vi "Puff_Dose.vi"() -> (5 "Plug in titles":string[](array[string]), 7 "Plug in values":string[](array[string]))   [LabVIEW 2015]
uses:
  Controls/Post_Process.ctl
  <vilib>/Analysis/baseanly.llb/Mean (DBL).vi
  Globals/Meas_global.vi
  Globals/Plug_in_data_global.vi
  <vilib>/Analysis/NI_AALBase.lvlib
panel:
  out "Active Trace length":i32
  out "Background time used (s)":dbl
  out "Delta T":dbl
  out "Min Dose":dbl
  out "Stats Names":string[](array[string])
  out "Stats values":string[](array[string])
  in  "File Extension":string=".xls"
  in  "Save Puff file":bool
  out "Bkgnd value (ppm)":dbl format="%0.2f"
  out "Array":dbl[][](array[numeric])
  out "Puff Number":i32=51
  out "XY Graph":cluster{"Time (s)":dbl[], "Eng Values":dbl[]}[](graph)
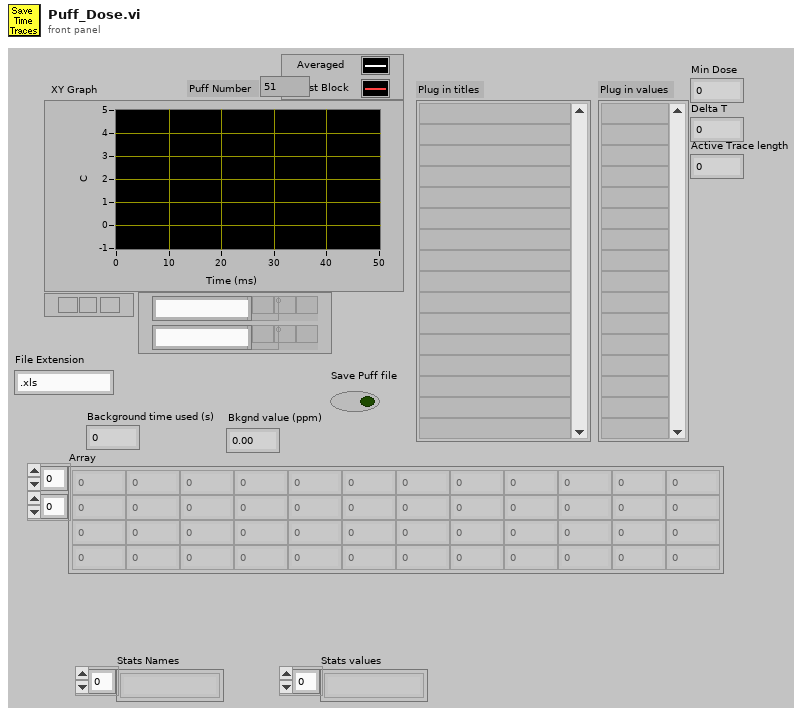
[diagram p1: front panel]
types:
  T1 = typedef "Analysis_info_cluster.ctl" = cluster{"Colour":u32, "Inst type":T2, "Inst name":string, "Symbol":string, "Code name":string, "Extra Info":string, "Inst Array":T3, "Extra Titles":string[], "Extra Values":string[], "U":dbl, "u^2":dbl, "u^3":dbl, "u^4":dbl, "Skew_u":dbl, "Kurt_u":dbl, "Sd Error in Mean":dbl, "% u'/U":dbl, "X":dbl, "Y":dbl, "Z":dbl, "Timescale integral to 25%":dbl, "Sd Error in Variance":dbl, "Calib File":path, "Calib Constants":dbl[], "Output Position":bool, "Full Stats":bool, "Av Sampling Rate":dbl, "Av No of Samples":dbl, "Total Meas Time (s)":dbl, "ADAM Ch Name":string}
  T2 = typedef "Inst_type.ctl" = enum16{"Propeller anemometer", "Raw voltage", "Pressure Transducer", "Pitot-static tube", "Preston tube", "Hot wire", "Cross wire 1", "Cross wire 2", "Generic Linear", "Generic Polynomial", "Generic BackPoly", "Fast FID", "Thermocouple", "Cold wire", "Pulsed Wire", "LDA Vel", "LDA Tran time", "LDA Arr time", "Microphone"}
  T3 = typedef "Instrument_Array.ctl" = enum16{"PWA", "LDA", "Analogue"}
  T4 = typedef "Post_Process.ctl" = enum16{"Take New Data", "Post Process Raw Data File"}
  T5 = enum16{"Save no data", "Save data in new files", "Save data in existing files"}
  T6 = typedef "Time_Trace_Cluster.ctl" = cluster{"Weighting":dbl[], "Time (s)":dbl[], "Voltage":dbl[], "Eng Values":dbl[]}
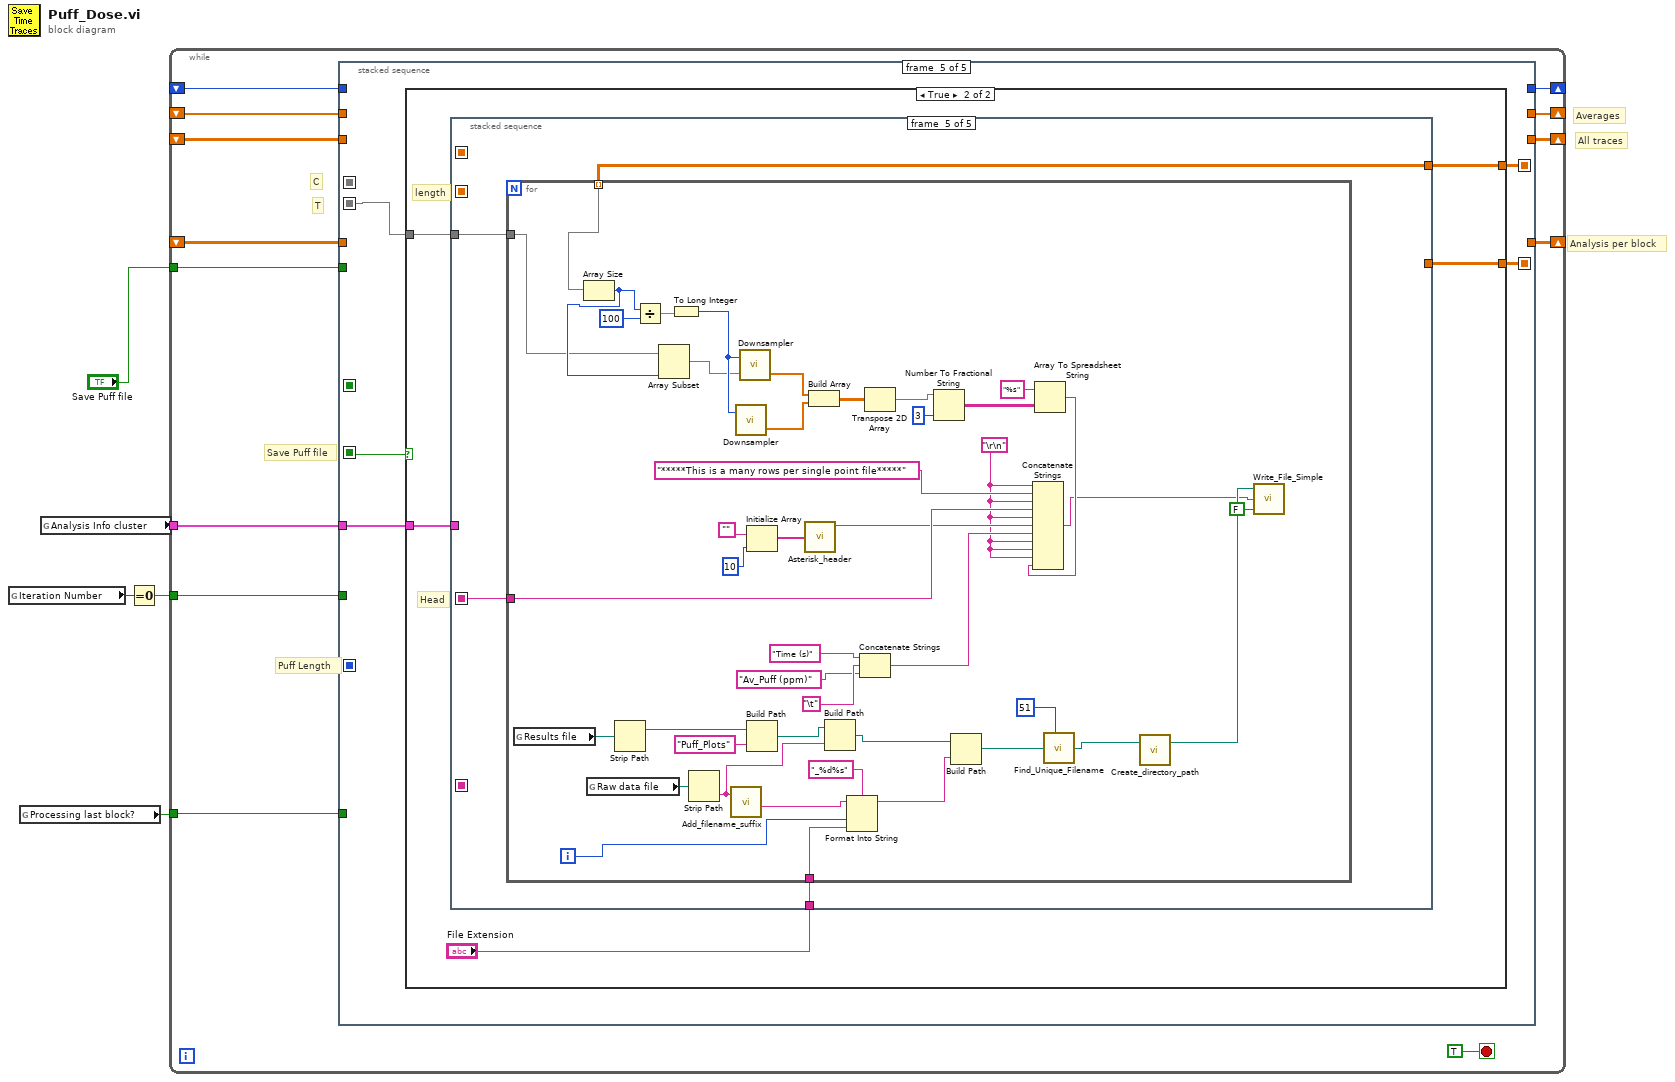
[diagram p0: block diagram]
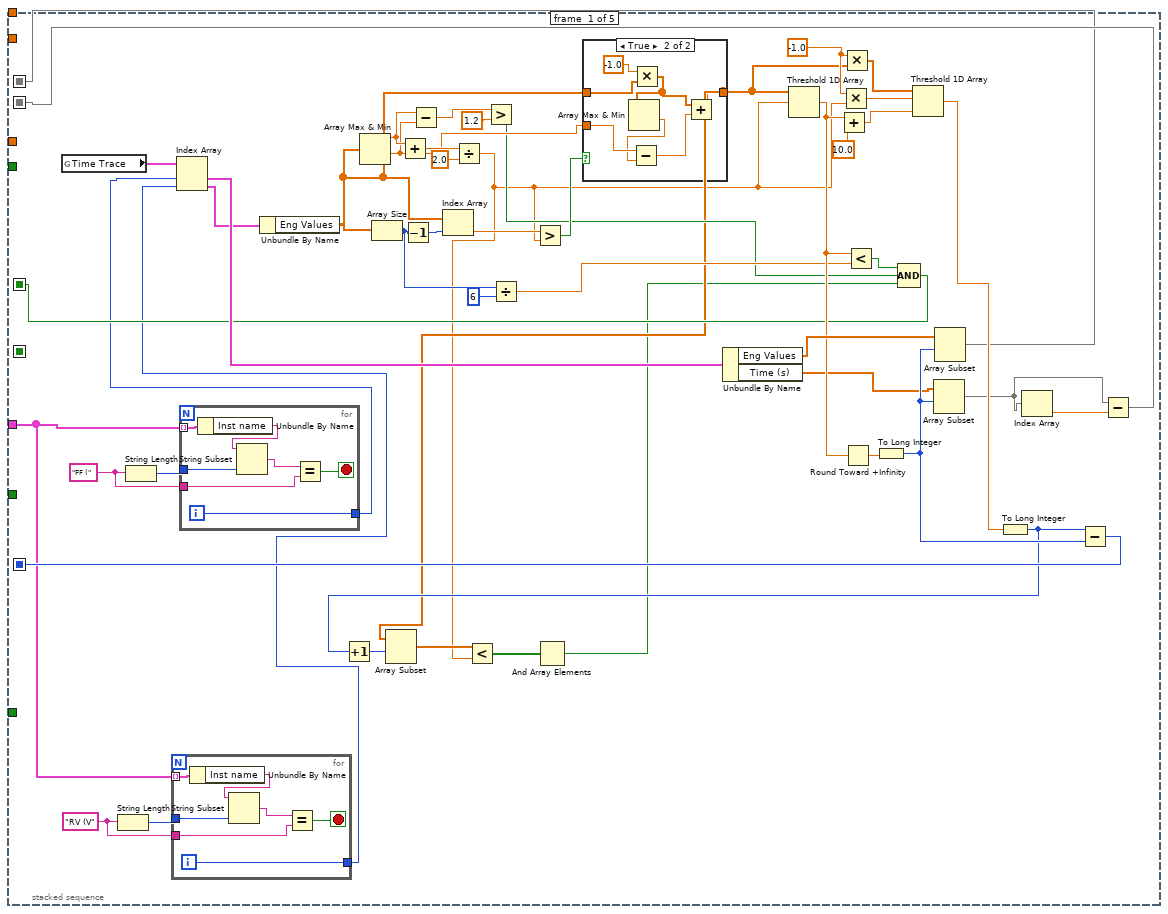
[diagram p2: hidden frame]
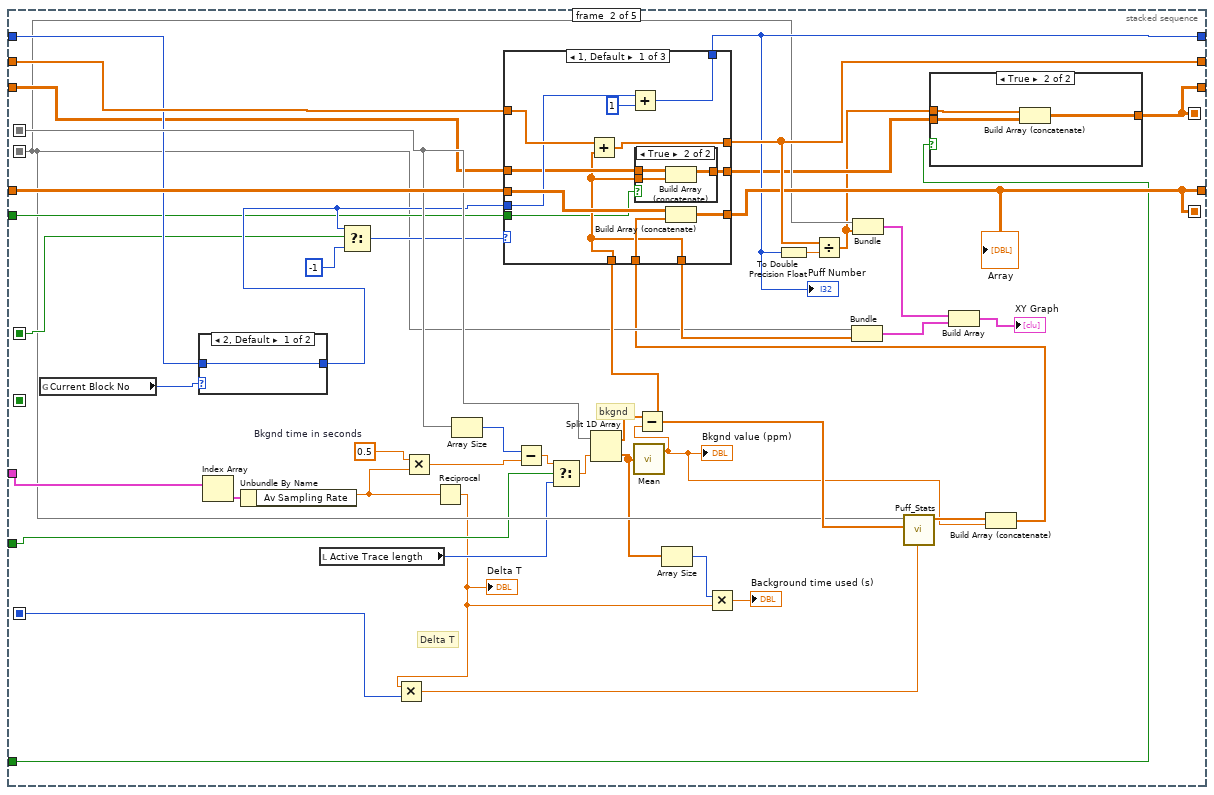
[diagram p4: hidden frame]
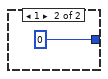
[diagram p6: hidden frame]
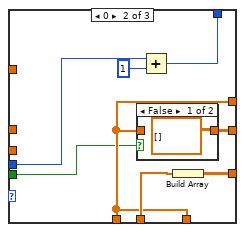
[diagram p8: hidden frame]
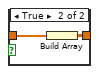
[diagram p9: hidden frame]
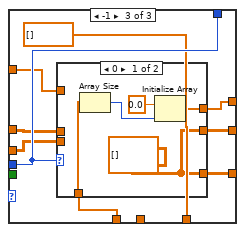
[diagram p10: hidden frame]
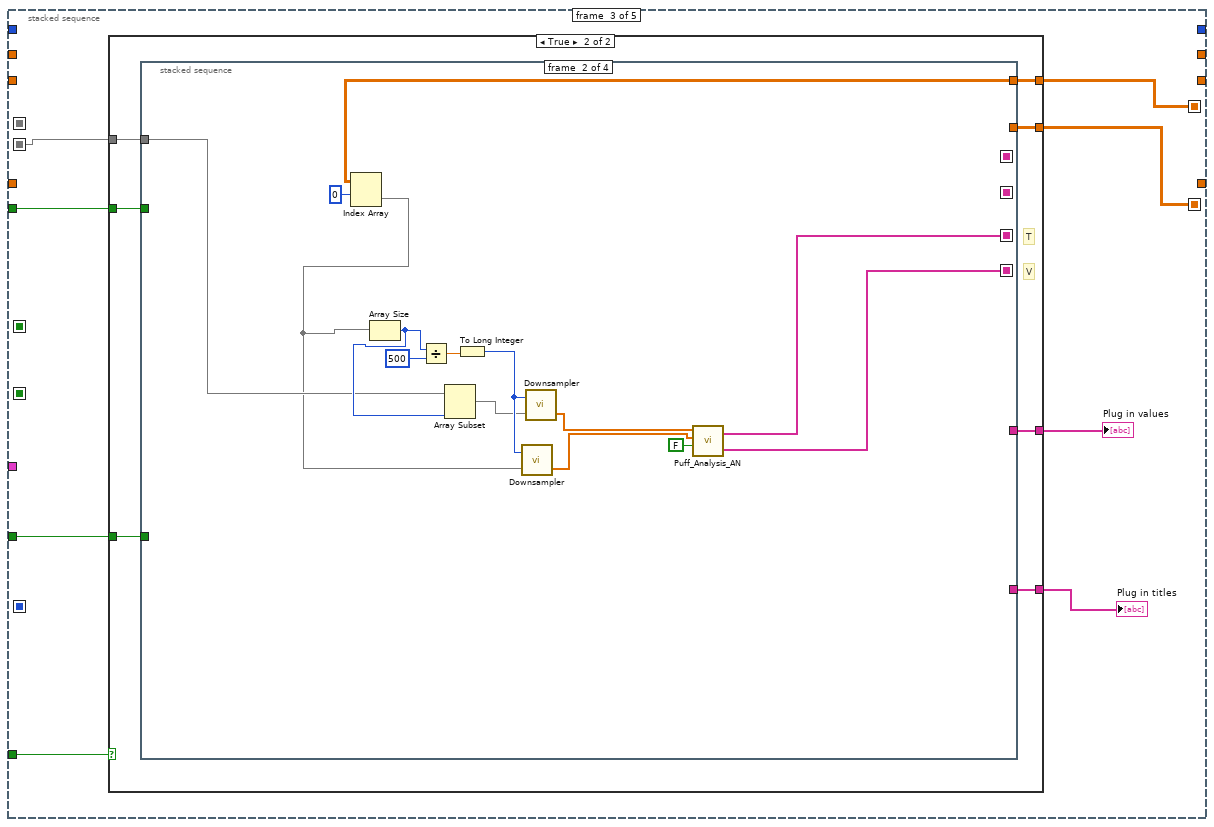
[diagram p12: hidden frame]
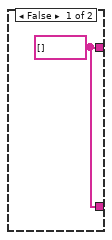
[diagram p13: hidden frame]
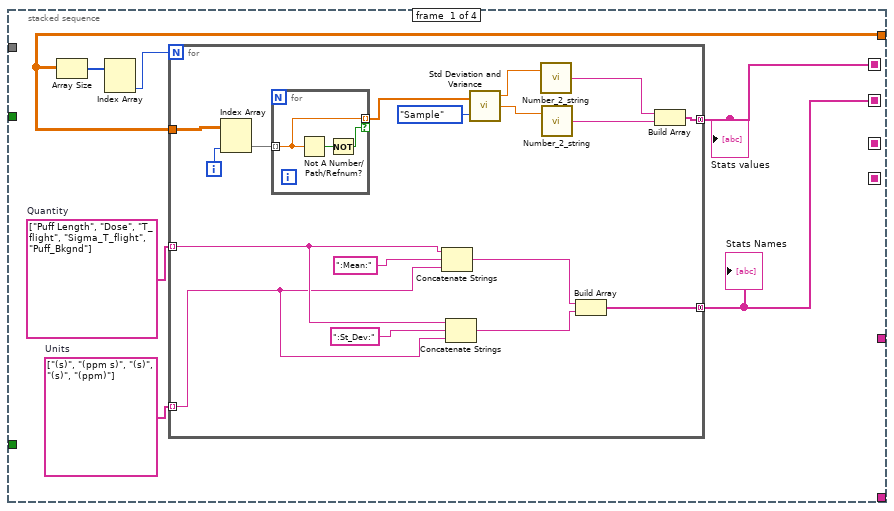
[diagram p14: hidden frame]
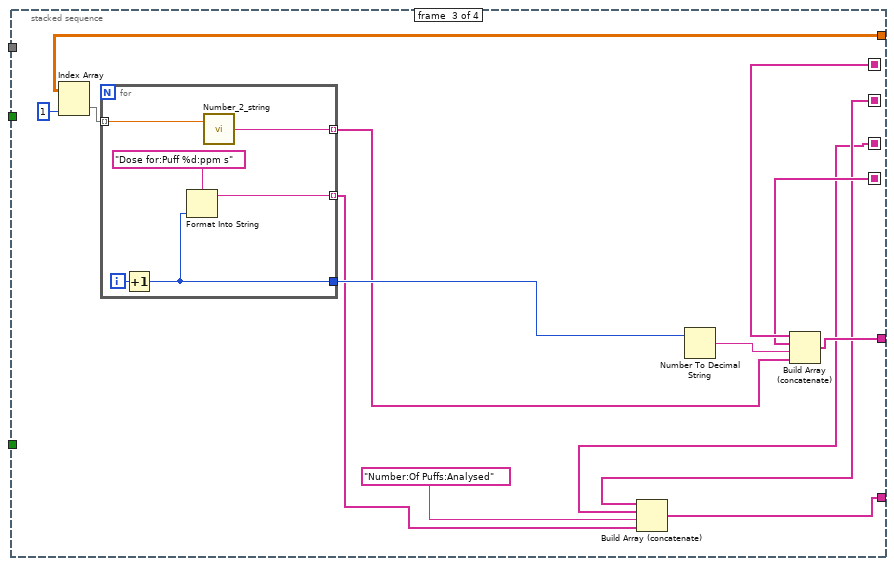
[diagram p15: hidden frame]
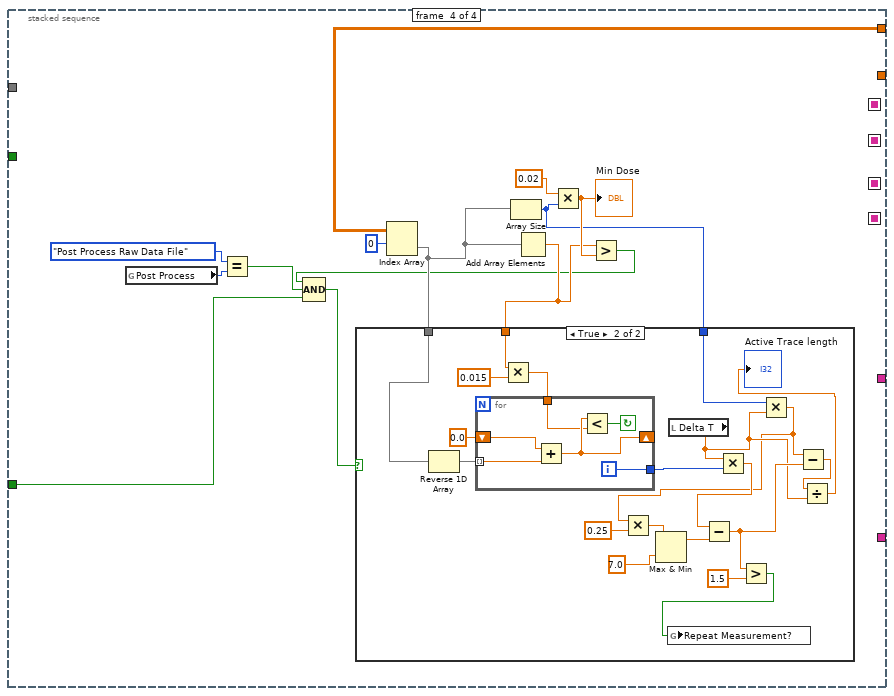
[diagram p16: hidden frame]
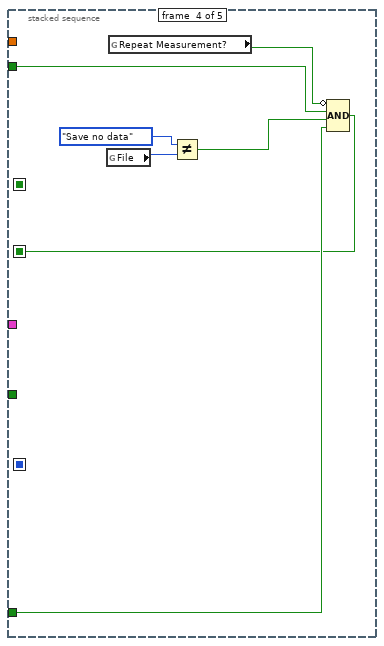
[diagram p18: hidden frame]
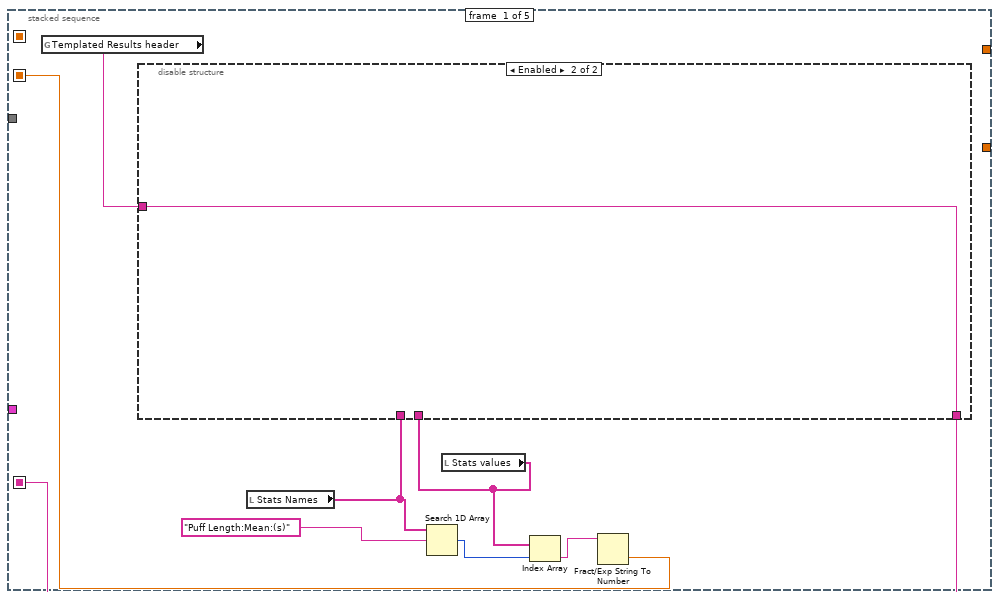
[diagram p20: hidden frame]
diagram:
  # "Averages"
  # "All traces"
  # "Analysis per block"
  n1 = global read "Meas_global.vi" "Iteration Number"() -> (w2:i32)
  n2 = global read "Meas_global.vi" "Processing last block?"() -> (w3:bool)
  n3 = global read "Meas_global.vi" "Analysis Info cluster"() -> (w5:T1[])
  n4 = Equal To 0?(x=w2) -> (x = 0?=w1:bool)
  n5 = while {
    shift-right: [w16] -> _
    shift-left: _ -> [w18]
    shift-right: [w14] -> _
    shift-left: _ -> [w15]
    tunnel: w5 -> [w13]
    shift-right: [w11] -> _
    shift-left: _ -> [w12]
    shift-right: [w10] -> _
    shift-left: _ -> [w9]
    tunnel: "Save Puff file" -> [w8]
    tunnel: w3 -> [w7]
    tunnel: w1 -> [w6]
    stop <- TRUE stop-if-true
    # "Save Puff file"
    # "Puff Length"
    # "T"
    # "C"
    n6 = stacked-sequence {
      seq-local: [_ w123 _ _ _] -> [_ _ w192 _ w311]
      seq-local: [w34 _ _ _ _] -> [_ w122 _ _ _]
      seq-local: [w35 _ _ _ _] -> [_ w106 w185 _ w309]
      seq-local: [w33 _ _ _ _] -> [_ w120 _ _ _]
      seq-local: [w38 _ _ _ _] -> [_ w112 _ _ _]
      seq-local: [_ w102 _ _ _] -> [_ _ w186 _ w312]
      seq-local: [_ _ _ w302 _] -> [_ _ _ _ w308]
      tunnel: w18 -> [_ w119 _ _ _]
      tunnel: [_ w133 _ _ _] -> w16
      tunnel: w15 -> [_ w124 _ _ _]
      tunnel: [_ w123 _ _ _] -> w14
      tunnel: w13 -> [w21 w121 _ _ w310]
      tunnel: w12 -> [_ w117 _ _ _]
      tunnel: [_ w116 _ _ _] -> w11
      tunnel: [_ w102 _ _ _] -> w10
      tunnel: w9 -> [_ w108 _ _ _]
      tunnel: w8 -> [_ w107 w189 w305 _]
      tunnel: w7 -> [_ w105 w188 w303 _]
      tunnel: w6 -> [_ w99 w187 _ _]
      frame #0 {
        w23 = "RV (V"
        w58 = -1.0
        w65 = "FF ("
        n7 = global read "Meas_global.vi" "Time Trace"() -> (w67:T6[])
        n8 = String Length(string=w23) -> (length=w22:i32)
        n9 = String Length(string=w65) -> (length=w66:i32)
        n10 = for {
          tunnel: w21 -> [w74] mode=indexing
          tunnel: w22 -> [w73]
          tunnel: w23 -> [w70]
          tunnel: [w68] -> w20
          i -> [w68]
          stop <- w69 stop-if-true
          n11 = Unbundle By Name(w74) -> ("Inst name"=w72:string)
          n12 = String Subset(string=w72, length (rest)=w73) -> (substring=w71:string)  [unwired: 1 in]
          n13 = Equal?(x=w71, y=w70) -> (x = y?=w69:bool)
        }
        n14 = for {
          tunnel: w21 -> [w89] mode=indexing
          tunnel: w66 -> [w88]
          tunnel: w65 -> [w85]
          tunnel: [w83] -> w19
          i -> [w83]
          stop <- w84 stop-if-true
          n15 = Unbundle By Name(w89) -> ("Inst name"=w87:string)
          n16 = String Subset(string=w87, length (rest)=w88) -> (substring=w86:string)  [unwired: 1 in]
          n17 = Equal?(x=w86, y=w85) -> (x = y?=w84:bool)
        }
        n18 = Index Array(array=w67, index #1=w19, index #2=w20) -> (element #1=w64:T6, element #2=w63:T6)
        n19 = Unbundle By Name(w63) -> ("Eng Values"=w30:dbl[])
        n20 = Array Max & Min(array=w30) -> (max value=w48:dbl, min value=w47:dbl)  [unwired: 2 out]
        n21 = Array Size(array=w30) -> (size(s)=w43:i32)
        n22 = Add(x=w48, y=w47) -> (x+y=w62:dbl)
        n23 = Decrement(x=w43) -> (x-1=w52:i32)
        n24 = Subtract(x=w48, y=w47) -> (x-y=w46:dbl)
        n25 = Index Array(array=w30, index=w52) -> (element=w51:dbl)
        n26 = Divide(x=w62, y=2.0) -> (x/y=w26:dbl)
        n27 = Greater?(x=w46, y=1.2) -> (0:w39:bool)
        n28 = Divide(x=w43, y=6) -> (x/y=w41:dbl)
        n29 = Greater?(x=w51, y=w26) -> (0:w50:bool)
        n30 = case shown="True" w50 {
          tunnel: w30 -> [w75 w81]
          tunnel: [w75 w76] -> w28
          tunnel: w47 -> [_ w80]
          frame False {
          }
          frame True {
            n31 = Multiply(x=-1.0, y=w81) -> (x*y=w77:dbl[])
            n32 = Array Max & Min(array=w77) -> (min value=w79:dbl)  [unwired: 3 out]
            n33 = Subtract(x=w80, y=w79) -> (x-y=w78:dbl)
            n34 = Add(x=w77, y=w78) -> (x+y=w76:dbl[])
          }
        }
        n35 = Unbundle By Name(w64) -> ("Eng Values"=w55:dbl[], "Time (s)"=w31:dbl[])
        n36 = Threshold 1D Array(2:w26, 3:w28) -> (0:w44:dbl)  [unwired: 1 in]
        n37 = Add(x=w44, y=10.0) -> (x+y=w60:dbl)
        n38 = Multiply(x=w58, y=w26) -> (x*y=w57:dbl)
        n39 = Multiply(x=w58, y=w28) -> (x*y=w49:dbl[])
        n40 = Round Toward +Infinity(x=w44) -> (ceil(x): smallest int >= x=w56:dbl)
        n41 = Less?(x=w44, y=w41) -> (x < y?=w40:bool)
        n42 = To Long Integer(number=w56) -> (32bit integer=w53:i32)
        n43 = Threshold 1D Array(1:w60, 2:w57, 3:w49) -> (0:w54:dbl)
        n44 = Array Subset(array=w31, index=w53) -> (w36:dbl[])  [unwired: 1 in]
        n45 = Array Subset(array=w55, index=w53) -> (w34:dbl[])  [unwired: 1 in]
        n46 = To Long Integer(number=w54) -> (32bit integer=w32:i32)
        n47 = Increment(x=w32) -> (x+1=w29:i32)
        n48 = Array Subset(array=w28, index=w29) -> (w27:dbl[])  [unwired: 1 in]
        n49 = Less?(x=w27, y=w26) -> (x < y?=w25:bool[])
        n50 = And Array Elements(Boolean array=w25) -> (logical AND=w24:bool)
        n51 = Compound Arithmetic op=AND(w40, w39, w24) -> (w38:bool)
        n52 = Index Array(array=w36) -> (element=w37:dbl)  [unwired: 1 in]
        n53 = Subtract(x=w32, y=w53) -> (x-y=w33:i32)
        n54 = Subtract(x=w36, y=w37) -> (x-y=w35:dbl[])
      }
      frame #1 {
        w94 = 0.5  # Bkgnd time in seconds
        # "bkgnd"
        # "Delta T"
        n55 = global read "Meas_global.vi" "Current Block No"() -> (w118:i32)
        n56 = case shown="2, Default" w118 {
          tunnel: [w139 0] -> w115
          tunnel: w117 -> [w139 _]
          frame 2, Default {
          }
          frame 1 {
          }
        }
        n57 = Index Array(array=w121) -> (element=w129:T1)  [unwired: 1 in]
        n58 = Unbundle By Name(w129) -> ("Av Sampling Rate"=w125:dbl)
        n59 = local read "Active Trace length"() -> (w98:i32)
        n60 = Select(t=w115, s=w112, f=-1) -> (s? t:f=w113:i32)
        n61 = Multiply(x=w94, y=w125) -> (x*y=w127:dbl)
        n62 = Reciprocal(x=w125) -> (1/x=w95:dbl)
        "Delta T" <- w95
        n63 = Multiply(x=w95, y=w120) -> (x*y=w111:dbl)
        n64 = Array Size(array=w122) -> (size(s)=w128:i32)
        n65 = Subtract(x=w128, y=w127) -> (x-y=w101:dbl)
        n66 = Select(t=w101, s=w99, f=w98) -> (s? t:f=w100:dbl)
        n67 = Split 1D Array(array=w122, index=w100) -> (first subarray=w126:dbl[], second subarray=w97:dbl[])
        n68 = call-poly <vilib>:"Mean.vi"("X"=w97) -> ("mean"=w90:dbl)  [unwired: 1 out]
        "Bkgnd value (ppm)" <- w90
        n69 = Subtract(x=w126, y=w90) -> (x-y=w110:dbl[])
        n70 = Array Size(array=w97) -> (size(s)=w96:i32)
        n71 = Multiply(x=w96, y=w95) -> (x*y=→"Background time used (s)":dbl)
        n72 = call "Puff_Stats.vi"("Puff release time (s)"=w111, "Concentrations"=w110, "Time (s)"=w106) -> ("Stats"=w93:dbl[])  [unwired: 8 in]
        n73 = Build Array (concatenate)(w93, w90) -> (w92:dbl[])
        n74 = case shown="1, Default" w113 {
          tunnel: [w151 w159 w175] -> w133
          tunnel: w119 -> [w152 _ w174]
          tunnel: w92 -> [w150 w164 _]
          tunnel: [w149 w163 w170] -> w123
          tunnel: w124 -> [w148 _ w173]
          tunnel: w115 -> [w145 w162 w176]
          tunnel: [w146 w160 w176] -> w116
          tunnel: w110 -> [w143 w159 w172]
          tunnel: [w143 w159 dbl[] []] -> w109
          tunnel: [w142 w158 w169] -> w104
          tunnel: w108 -> [w144 _ w168]
          tunnel: w107 -> [w141 w157 _]
          frame 1, Default {
            n75 = Add(x=w152, y=w143) -> (x+y=w151:dbl[])
            n76 = Add(x=w145, y=1) -> (x+y=w146:i32)
            n77 = case shown="True" w141 {
              tunnel: w144 -> [w153 w156]
              tunnel: w143 -> [_ w155]
              tunnel: [w153 w154] -> w142
              frame False {
              }
              frame True {
                n78 = Build Array (concatenate)(w156, w155) -> (w154:dbl[][])
              }
            }
            n79 = Build Array (concatenate)(w148, w150) -> (w149:dbl[][])
          }
          frame 0 {
            n80 = case shown="False" w157 {
              tunnel: w159 -> [_ w167]
              tunnel: [dbl[][] [] w166] -> w158
              frame False {
              }
              frame True {
                n81 = Build Array(w167) -> (w166:dbl[][])
              }
            }
            n82 = Add(x=w162, y=1) -> (x+y=w160:i32)
            n83 = Build Array(w164) -> (w163:dbl[][])
          }
          frame -1 {
            n84 = case shown="0" w176 {
              tunnel: w172 -> [w181 _]
              tunnel: [w178 w184] -> w175
              tunnel: [w177 w183] -> w170
              tunnel: w174 -> [_ w184]
              tunnel: w173 -> [_ w183]
              tunnel: [w177 w182] -> w169
              tunnel: w168 -> [_ w182]
              frame 0 {
                w177 = dbl[][] []
                n85 = Array Size(array=w181) -> (size(s)=w180:i32)
                n86 = Initialize Array(0.0 ("element"), w180) -> (w178:dbl[])
              }
              frame 1, Default {
              }
            }
          }
        }
        "Puff Number" <- w116
        "Array" <- w123
        n87 = To Double Precision Float(number=w116) -> (double precision float=w134:dbl)
        n88 = Divide(x=w133, y=w134) -> (x/y=w103:dbl[])
        n89 = Bundle(w106, w109) -> (w132:cluster{dbl[], dbl[]})  [unwired: 1 in]
        n90 = Bundle(w106, w103) -> (w131:cluster{dbl[], dbl[]})  [unwired: 1 in]
        n91 = case shown="True" w105 {
          tunnel: w104 -> [w135 w138]
          tunnel: w103 -> [_ w137]
          tunnel: [w135 w136] -> w102
          frame False {
          }
          frame True {
            n92 = Build Array (concatenate)(w137, w138) -> (w136:dbl[][])
          }
        }
        n93 = Build Array(w131, w132) -> (→"XY Graph":cluster{dbl[], dbl[]}[])
      }
      frame #2 {
        n94 = case shown="True" w188 {
          tunnel: w192 -> [_ w200]
          tunnel: [w193 w199] -> w191
          tunnel: [w193 w198] -> w190
          tunnel: w189 -> [_ w197]
          tunnel: w187 -> [_ w196]
          tunnel: w186 -> [_ w195]
          tunnel: w185 -> [_ w194]
          frame False {
            w193 = string[] []
          }
          frame True {
            # "T"
            # "V"
            n95 = stacked-sequence {
              seq-local: [w202 _ _ _] -> [_ _ w250 _]
              seq-local: [w201 _ _ _] -> [_ _ w243 _]
              seq-local: [_ w229 _ _] -> [_ _ w242 _]
              seq-local: [_ w228 _ _] -> [_ _ w244 _]
              tunnel: w200 -> [w205 _ w253 _]
              tunnel: [_ _ w255 _] -> w199
              tunnel: [_ _ w254 _] -> w198
              tunnel: w197 -> [_ _ _ _]
              tunnel: w196 -> [_ _ _ w271]
              tunnel: w195 -> [_ w240 _ w270]
              tunnel: w194 -> [_ w234 _ _]
              frame #0 {
                w203 = string[] ["(s)", "(ppm s)", "(s)", "(s)", "(ppm)"]  # Units
                w204 = string[] ["Puff Length", "Dose", "T_flight", "Sigma_T_flight", "Puff_Bkgnd"]  # Quantity
                n96 = Array Size(array=w205) -> (size(s)=w207:i32[])
                n97 = Index Array(array=w207) -> (element #2=w206:i32)  [unwired: 2 in, 1 out]
                n98 = for {
                  N: w206 -> [_]
                  tunnel: w205 -> [w224]
                  tunnel: w204 -> [w215] mode=indexing
                  tunnel: w203 -> [w214] mode=indexing
                  tunnel: [w211] -> w202 mode=concatenating
                  tunnel: [w210] -> w201 mode=concatenating
                  i -> [w223]
                  n99 = Index Array(array=w224, index (col)=w223) -> (element=w209:dbl[])  [unwired: 1 in]
                  n100 = for {
                    tunnel: w209 -> [w227] mode=indexing
                    tunnel: [w227] -> w208 mode=indexing if=w225
                    n101 = Not A Number/Path/Refnum?(number/path/refnum=w227) -> (NaN/Path/Refnum?=w226:bool)
                    n102 = Not(x=w226) -> (.not. x?=w225:bool)
                  }
                  n103 = Concatenate Strings(w215, ":Mean:" ("string"), w214) -> (w212:string)
                  n104 = Concatenate Strings(w215, ":St_Dev:" ("string"), w214) -> (w213:string)
                  n105 = call <vilib>:"Std Deviation and Variance.vi"("X"=w208, "Weighting (Sample)"=enum16{"Sample", "Population"}."Sample") -> ("mean"=w220:dbl, "standard deviation"=w221:dbl)  [unwired: 1 out]
                  n106 = call "Number_2_string.vi"("number"=w220) -> ("String"=w219:string)  [unwired: 1 in]
                  n107 = call "Number_2_string.vi"("number"=w221) -> ("String"=w218:string)  [unwired: 1 in]
                  n108 = Build Array(w212, w213) -> (w210:string[])
                  n109 = Build Array(w219, w218) -> (w211:string[])
                }
                "Stats values" <- w202
                "Stats Names" <- w201
              }
              frame #1 {
                n110 = Index Array(array=w240, index (row)=0) -> (element=w232:dbl[])  [unwired: 1 in]
                n111 = Array Size(array=w232) -> (size(s)=w235:i32)
                n112 = Divide(x=w235, y=500) -> (x/y=w237:dbl)
                n113 = Array Subset(array=w234, length=w235) -> (w233:dbl[])  [unwired: 1 in]
                n114 = To Long Integer(number=w237) -> (32bit integer=w236:i32)
                n115 = call "Downsampler.vi"("Input Array"=w232, "Averaging samples"=w236) -> ("Downsampled Array"=w230:dbl[])  [unwired: 1 out]
                n116 = call "Downsampler.vi"("Input Array"=w233, "Averaging samples"=w236) -> ("Downsampled Array"=w231:dbl[])  [unwired: 1 out]
                n117 = call "Puff_Analysis_AN.vi"("Input Own Peak Value?"=FALSE, "Concentration"=w230, "Time"=w231) -> ("Channel Values"=w228:string[], "Channel Names"=w229:string[])  [unwired: 3 in]
              }
              frame #2 {
                n118 = Index Array(array=w253, index (col)=1 ("disabled index (col)")) -> (element=w251:dbl[])  [unwired: 1 in]
                n119 = for {
                  tunnel: w251 -> [w261] mode=indexing
                  tunnel: [w258] -> w247 mode=indexing
                  tunnel: [w257] -> w246 mode=indexing
                  tunnel: [w256] -> w249
                  i -> [w260]
                  n120 = Increment(x=w260) -> (x+1=w256:i32)
                  n121 = Format Into String(format string="Dose for:Puff %d:ppm s", w256) -> (resulting string=w257:string)  [unwired: 2 in, 1 out]
                  n122 = call "Number_2_string.vi"("number"=w261) -> ("String"=w258:string)  [unwired: 1 in]
                }
                n123 = Build Array (concatenate)(w243, w242, "Number:Of Puffs:Analysed" ("format string"), w246) -> (w254:string[])
                n124 = Number To Decimal String(number=w249) -> (decimal integer string=w248:string)  [unwired: 1 in]
                n125 = Build Array (concatenate)(w250, w244, w248, w247) -> (w255:string[])
              }
              frame #3 {
                n126 = global read "Meas_global.vi" "Post Process"() -> (w274:T4)
                n127 = Equal?(x=Post_Process."Post Process Raw Data File" ("Post Process"), y=w274) -> (x = y?=w272:bool)
                n128 = Index Array(array=w270, index (row)=0) -> (element=w268:dbl[])  [unwired: 1 in]
                n129 = Array Size(array=w268) -> (size(s)=w262:i32)
                n130 = Add Array Elements(numeric array=w268) -> (sum=w265:dbl)
                n131 = Multiply(x=0.02, y=w262) -> (x*y=w266:dbl)
                "Min Dose" <- w266
                n132 = Greater?(x=w265, y=w266) -> (0:w264:bool)
                n133 = Compound Arithmetic op=AND(w264, w272, w271) -> (w263:bool)
                n134 = case shown="True" w263 {
                  tunnel: w268 -> [_ w292]
                  tunnel: w265 -> [_ w291]
                  tunnel: w262 -> [_ w284]
                  frame False {
                  }
                  frame True {
                    n135 = Reverse 1D Array(array=w292) -> (reversed array=w294:dbl[])
                    n136 = Multiply(x=w291, y=0.015) -> (x*y=w289:dbl)
                    n137 = for {
                      shift-right: [w298] -> _
                      shift-left: 0.0 -> [w299]
                      tunnel: w294 -> [w300] mode=indexing
                      tunnel: w289 -> [w297]
                      tunnel: [w295] -> w285
                      i -> [w295]
                      stop <- w296 continue-if-true
                      n138 = Add(x=w299, y=w300) -> (x+y=w298:dbl)
                      n139 = Less?(x=w298, y=w297) -> (x < y?=w296:bool)
                    }
                    n140 = local read "Delta T"() -> (w281:dbl)
                    n141 = Multiply(x=w281, y=w285) -> (x*y=w288:dbl)
                    n142 = Multiply(x=w284, y=w281) -> (x*y=w279:dbl)
                    n143 = Multiply(x=w279, y=0.25) -> (x*y=w277:dbl)
                    n144 = Max & Min(x=w277, y=7.0) -> (max(x,y)=w275:dbl)  [unwired: 1 out]
                    n145 = Subtract(x=w288, y=w275) -> (x-y=w283:dbl)
                    n146 = Greater?(x=w283, y=1.5) -> (0:w286:bool)
                    n147 = global write "Meas_global.vi" "Repeat Measurement?"(w286) -> ()
                    n148 = Subtract(x=w279, y=w283) -> (x-y=w282:dbl)
                    n149 = Divide(x=w282, y=w281) -> (x/y=→"Active Trace length":dbl)
                  }
                }
              }
            }
          }
        }
        "Plug in titles" <- w190
        "Plug in values" <- w191
      }
      frame #3 {
        n150 = global read "Meas_global.vi" "File"() -> (w307:T5)
        n151 = global read "Meas_global.vi" "Repeat Measurement?"() -> (w301:bool)
        n152 = Not Equal?(x=T5."Save no data" ("File"), y=w307) -> (x != y?=w304:bool)
        n153 = Compound Arithmetic op=AND(invert w301, w305, w304, w303) -> (w302:bool)
      }
      frame #4 {
        n154 = case shown="True" w308 {
          tunnel: w312 -> [_ w317]
          tunnel: w311 -> [_ w316]
          tunnel: w310 -> [_ w315]
          tunnel: w309 -> [_ w314]
          frame False {
          }
          frame True {
            # "Head"
            # "length"
            n155 = stacked-sequence {
              seq-local: [_ w388 _ _ _] -> [_ _ w423 _ _]
              seq-local: [w320 _ _ _ _] -> [_ _ w425 w475 w483]
              seq-local: [w322 _ _ _ _] -> [_ w376 _ _ _]
              seq-local: [_ w364 _ _ _] -> [_ _ _ w440 _]
              tunnel: w317 -> [_ w368 _ _ w480]
              tunnel: w316 -> [_ w374 _ _ _]
              tunnel: w315 -> [_ _ _ _ _]
              tunnel: w314 -> [_ w377 _ w441 w481]
              tunnel: "File Extension" -> [_ _ w421 w443 w482]
              frame #0 {
                n156 = global read "Plug_in_data_global.vi" "Templated Results header"() -> (w321:string)
                n157 = local read "Stats Names"() -> (w319:string[])
                n158 = Search 1D Array(1D array=w319, element="Puff Length:Mean:(s)") -> (index of element=w324:i32)  [unwired: 1 in]
                n159 = local read "Stats values"() -> (w318:string[])
                n160 = disable-structure shown="Enabled" {
                  disable-tunnel: w319 -> [w329 _]
                  disable-tunnel: w318 -> [w328 _]
                  disable-tunnel: w321 -> [w327 w363]
                  disable-tunnel: [w326 w363] -> w320
                  frame Disabled {
                    # "Add Puff Statistics if not in the template file\nHowever it channel name changes it adds it again!"
                    n161 = call "String_to_Ch_names.vi"("Spreadsheet string"=w327) -> ("Ch names"=w332:string[], "String After names"=w342:string)  [unwired: 2 out]
                    n162 = call "Split_at_return.vi"("String"=w342) -> ("before substring"=w343:string)  [unwired: 1 in, 3 out]
                    n163 = Spreadsheet String To Array(format string="%s", spreadsheet string=w343, array type (2D Dbl)=string[] [] ("Channel Values")) -> (array=w339:string[])  [unwired: 1 out]
                    n164 = for {
                      tunnel: w332 -> [w352]
                      tunnel: w329 -> [w351] mode=indexing
                      tunnel: [w350] -> w338 mode=indexing if=w345
                      tunnel: [w349] -> w337 mode=indexing if=w345
                      tunnel: w328 -> [w348] mode=indexing
                      shift-right: [w347] -> w336
                      shift-left: w339 -> [w346]
                      n165 = Search 1D Array(1D array=w352, element=w351) -> (index of element=w344:i32)  [unwired: 1 in]
                      n166 = case shown="-1" w344 {
                        tunnel: w351 -> [_ w362]
                        tunnel: [w357 w362] -> w350
                        tunnel: [w357 w361] -> w349
                        tunnel: w348 -> [w353 w361]
                        tunnel: [w354 w360] -> w347
                        tunnel: w346 -> [w355 w360]
                        tunnel: [FALSE TRUE] -> w345
                        tunnel: w344 -> [w356 _]
                        frame 0, Default {
                          w357 = ""
                          n167 = Replace Array Subset(array=w355, new element=w353, index=w356) -> (w354:string[])
                        }
                        frame -1 {
                        }
                      }
                    }
                    n168 = Build Array (concatenate)(w338, w332) -> (w334:string[])
                    n169 = Build Array (concatenate)(w337, w336) -> (w335:string[])
                    n170 = call "Ch_names_to_rows.vi"("Channel Names"=w334) -> ("3 Row names"=w333:string[][])
                    n171 = Build Array (concatenate)(w333, w335) -> (w330:string[][])
                    n172 = Array To Spreadsheet String(array=w330, 3:"%s" ("format string")) -> (spreadsheet string=w326:string)  [unwired: 1 in]
                  }
                  frame Enabled {
                  }
                }
                n173 = Index Array(array=w318, index=w324) -> (element=w323:string)
                n174 = Fract/Exp String To Number(string=w323) -> (number=w322:dbl)  [unwired: 3 in, 1 out]
              }
              frame #1 {
                w381 = ""
                n175 = Array Size(array=w368) -> (size(s)=w392:i32[])
                n176 = Index Array(array=w392) -> (element #1=w365:i32, element #2=w366:i32)  [unwired: 2 in]
                n177 = for {
                  N: w366 -> [_]
                  tunnel: w368 -> [w398]
                  tunnel: w365 -> [w396]
                  tunnel: [w395] -> w367 mode=indexing
                  i -> [w397]
                  n178 = for {
                    N: w396 -> [_]
                    tunnel: w398 -> [w407]
                    tunnel: w397 -> [w406]
                    tunnel: [w399] -> w395 mode=indexing
                    i -> [w405]
                    n179 = Index Array(array=w407, index (row)=w405, index (col)=w406) -> (element=w400:dbl)
                    n180 = Equal To 0?(x=w405) -> (x = 0?=w404:bool)
                    n181 = Select(t=i16 3, s=w404, f=i16 1 ("precision (6)")) -> (s? t:f=w401:i16)
                    n182 = Number To Fractional String(number=w400, precision (6)=w401) -> (F-format string=w399:string)  [unwired: 2 in]
                  }
                }
                n183 = for {
                  N: w366 -> [_]
                  tunnel: w377 -> [w412] mode=indexing
                  tunnel: [w411] -> w382 mode=indexing
                  n184 = call "Number_2_string.vi"("number"=w412) -> ("String"=w411:string)  [unwired: 1 in]
                }
                n185 = for {
                  N: w365 -> [_]
                  tunnel: [w415] -> w372 mode=indexing
                  tunnel: [""] -> w379 mode=indexing
                  i -> [w413]
                  n186 = Format Into String(format string="Puff_%d", w413) -> (resulting string=w415:string)  [unwired: 2 in, 1 out]
                }
                n187 = Index Array(array=w368, index (row)=0) -> (element=w364:dbl[])  [unwired: 1 in]
                n188 = Build Array (concatenate)(w381, "Puff_Length (s)", "Puff_Dose (ppm s)", "T_flight (s)", "Sigma_T_flight (s)", w381, "Time (s)", w382) -> (w391:string[])
                n189 = call "Puff_Stats.vi"("Puff release time (s)"=w376, "Concentrations"=w364, "Time (s)"=w377) -> ("Stats"=w375:dbl[])  [unwired: 8 in]
                n190 = Replace Array Subset(array=w372, new element="Averaged Puff", index=0) -> (w371:string[])
                n191 = Build Array (concatenate)(w375, w374) -> (w373:dbl[][])
                n192 = Transpose 2D Array(2D array=w373) -> (transposed array=w394:dbl[][])
                n193 = for {
                  tunnel: w394 -> [w418] mode=indexing
                  tunnel: [w417] -> w393 mode=indexing
                  n194 = for {
                    tunnel: w418 -> [w420] mode=indexing
                    tunnel: [w419] -> w417 mode=indexing
                    n195 = call "Number_2_string.vi"("number"=w420) -> ("String"=w419:string)  [unwired: 1 in]
                  }
                }
                n196 = Build Array (concatenate)(w371, w393, w379, w371, w367) -> (w390:string[][])
                n197 = for {
                  tunnel: w391 -> [w408] mode=indexing
                  tunnel: w390 -> [w410] mode=indexing
                  tunnel: [w409] -> w389 mode=indexing
                  n198 = Build Array (concatenate)(w408, w410) -> (w409:string[])
                }
                n199 = Array To Spreadsheet String(array=w389, 3:"%s" ("format string")) -> (spreadsheet string=w388:string)  [unwired: 1 in]
              }
              frame #2 {
                w424 = "\r\n"
                n200 = global read "Meas_global.vi" "Results file"() -> (w438:path)
                n201 = Strip Path(path=w438) -> (stripped path=w437:path)  [unwired: 1 out]
                n202 = global read "Meas_global.vi" "Raw data file"() -> (w434:path)
                n203 = Strip Path(path=w434) -> (name=w435:string)  [unwired: 1 out]
                n204 = Build Path(base path=w437, name or relative path="Puff_Analysis") -> (appended path=w433:path)
                n205 = call "Add_filename_suffix.vi"("Filename"=w435) -> ("Base name"=w432:string)  [unwired: 1 in, 3 out]
                n206 = Concatenate Strings(w432, w421) -> (w431:string)
                n207 = Build Path(base path=w433, name or relative path=w431) -> (appended path=w430:path)
                n208 = Concatenate Strings(w425, w424, w424, w423) -> (w422:string)
                n209 = call "Find_Unique_Filename.vi"("Path In"=w430, "Max Length (31)"=51) -> ("Unique Path Out"=w428:path)  [unwired: 1 in]
                n210 = call "Create_directory_path.vi"("Path name"=w428) -> ("Path name Out"=w427:path)  [unwired: 1 in, 1 out]
                n211 = call "Write_File_Simple.vi"("append to file? (new file:F)"=FALSE, "character string"=w422, "file path"=w427) -> ()  [unwired: 2 out]
              }
              frame #3 {
                w459 = "\r\n"
                n212 = global read "Meas_global.vi" "Results file"() -> (w457:path)
                n213 = Array Size(array=w440) -> (size(s)=w442:i32)
                n214 = Divide(x=w442, y=100) -> (x/y=w478:dbl)
                n215 = Array Subset(array=w441, length=w442) -> (w439:dbl[])  [unwired: 1 in]
                n216 = Strip Path(path=w457) -> (stripped path=w456:path)  [unwired: 1 out]
                n217 = To Long Integer(number=w478) -> (32bit integer=w477:i32)
                n218 = global read "Meas_global.vi" "Raw data file"() -> (w453:path)
                n219 = call "Downsampler.vi"("Input Array"=w440, "Averaging samples"=w477) -> ("Downsampled Array"=w465:dbl[])  [unwired: 1 out]
                n220 = call "Downsampler.vi"("Input Array"=w439, "Averaging samples"=w477) -> ("Downsampled Array"=w466:dbl[])  [unwired: 1 out]
                n221 = Strip Path(path=w453) -> (name=w454:string)  [unwired: 1 out]
                n222 = Initialize Array("", 10) -> (w472:string[])
                n223 = Build Path(base path=w456, name or relative path="Av_Puff_Plots") -> (appended path=w452:path)
                n224 = Build Array(w466, w465) -> (w464:dbl[][])
                n225 = call "Add_filename_suffix.vi"("Filename"=w454) -> ("Base name"=w451:string)  [unwired: 1 in, 3 out]
                n226 = call "Asterisk_header.vi"("Channel names"=w472) -> ("Header string"=w471:string)
                n227 = Transpose 2D Array(2D array=w464) -> (transposed array=w462:dbl[][])
                n228 = Concatenate Strings(w451, w443) -> (w450:string)
                n229 = Concatenate Strings("Time (s)", "\t", "Av_Puff (ppm)") -> (w467:string)
                n230 = Number To Fractional String(number=w462, precision (6)=i16 3) -> (F-format string=w460:string[][])  [unwired: 2 in]
                n231 = Build Path(base path=w452, name or relative path=w450) -> (appended path=w449:path)
                n232 = Array To Spreadsheet String(array=w460, 3:"%s" ("format string")) -> (spreadsheet string=w458:string)  [unwired: 1 in]
                n233 = Concatenate Strings(w459, "*****This is a many rows per single point file*****", w459, w475, w459, w471, w467, w459, w459, w459, w458) -> (w444:string)
                n234 = call "Find_Unique_Filename.vi"("Path In"=w449, "Max Length (31)"=51) -> ("Unique Path Out"=w447:path)  [unwired: 1 in]
                n235 = call "Create_directory_path.vi"("Path name"=w447) -> ("Path name Out"=w446:path)  [unwired: 1 in, 1 out]
                n236 = call "Write_File_Simple.vi"("append to file? (new file:F)"=FALSE, "character string"=w444, "file path"=w446) -> ()  [unwired: 2 out]
              }
              frame #4 {
                n237 = for {
                  tunnel: w483 -> [w523]
                  tunnel: w482 -> [w492]
                  tunnel: w481 -> [w494]
                  tunnel: w480 -> [w484] mode=indexing
                  i -> [w491]
                  w507 = "\r\n"
                  n238 = global read "Meas_global.vi" "Results file"() -> (w505:path)
                  n239 = Array Size(array=w484) -> (size(s)=w495:i32)
                  n240 = global read "Meas_global.vi" "Raw data file"() -> (w502:path)
                  n241 = Strip Path(path=w505) -> (stripped path=w504:path)  [unwired: 1 out]
                  n242 = Divide(x=w495, y=100) -> (x/y=w526:dbl)
                  n243 = Array Subset(array=w494, length=w495) -> (w493:dbl[])  [unwired: 1 in]
                  n244 = To Long Integer(number=w526) -> (32bit integer=w525:i32)
                  n245 = Strip Path(path=w502) -> (name=w486:string)  [unwired: 1 out]
                  n246 = call "Add_filename_suffix.vi"("Filename"=w486) -> ("Base name"=w490:string)  [unwired: 1 in, 3 out]
                  n247 = call "Downsampler.vi"("Averaging samples"=w525) -> ("Downsampled Array"=w513:dbl[])  [unwired: 1 in, 1 out]
                  n248 = call "Downsampler.vi"("Input Array"=w493, "Averaging samples"=w525) -> ("Downsampled Array"=w514:dbl[])  [unwired: 1 out]
                  n249 = Initialize Array("", 10) -> (w520:string[])
                  n250 = Build Path(base path=w504, name or relative path="Puff_Plots") -> (appended path=w487:path)
                  n251 = call "Asterisk_header.vi"("Channel names"=w520) -> ("Header string"=w519:string)
                  n252 = Build Array(w514, w513) -> (w512:dbl[][])
                  n253 = Build Path(base path=w487, name or relative path=w486) -> (appended path=w485:path)
                  n254 = Format Into String(format string="_%d%s", initial string=w490, w491, w492) -> (resulting string=w489:string)  [unwired: 1 in, 1 out]
                  n255 = Concatenate Strings("Time (s)", "\t", "Av_Puff (ppm)") -> (w515:string)
                  n256 = Transpose 2D Array(2D array=w512) -> (transposed array=w510:dbl[][])
                  n257 = Number To Fractional String(number=w510, precision (6)=i16 3) -> (F-format string=w508:string[][])  [unwired: 2 in]
                  n258 = Build Path(base path=w485, name or relative path=w489) -> (appended path=w501:path)
                  n259 = Array To Spreadsheet String(array=w508, 3:"%s" ("format string")) -> (spreadsheet string=w506:string)  [unwired: 1 in]
                  n260 = Concatenate Strings(w507, "*****This is a many rows per single point file*****", w507, w523, w507, w519, w515, w507, w507, w507, w506) -> (w496:string)
                  n261 = call "Find_Unique_Filename.vi"("Path In"=w501, "Max Length (31)"=51) -> ("Unique Path Out"=w499:path)  [unwired: 1 in]
                  n262 = call "Create_directory_path.vi"("Path name"=w499) -> ("Path name Out"=w498:path)  [unwired: 1 in, 1 out]
                  n263 = call "Write_File_Simple.vi"("append to file? (new file:F)"=FALSE, "character string"=w496, "file path"=w498) -> ()  [unwired: 2 out]
                }
              }
            }
          }
        }
      }
    }
  }
